vi "Write Lines.vi"(8 "error in (no error)":errorcluster, 10 "Lines":T1[](array[typedef]), 11 "J1939 configuration in":refnum<class "J1939 configuration.lvclass">) -> (0 "error out":errorcluster, 3 "J1939 configuration out":refnum<class "J1939 configuration.lvclass">)   [LabVIEW 2014, in "J1939 configuration.lvclass"]
uses:
  J1939 configuration.lvclass
  Line.ctl
  <vilib>/NI/Tag Bus Module Framework/channel/TBM channel.lvclass
  J1939 configuration.lvclass/J1939 configuration.ctl
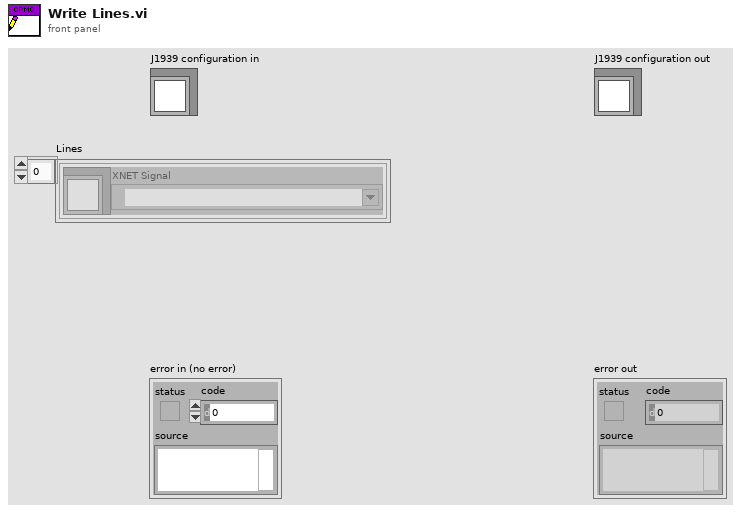
[diagram p1: front panel]
types:
  T1 = typedef "J1939 configuration.lvclass/Line.ctl" = cluster{"channel":refnum<class "TBM channel.lvclass">, "XNET Signal":refnum<k21>}
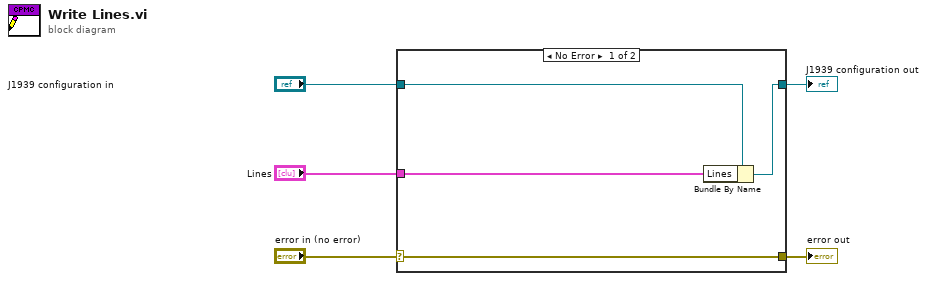
[diagram p0: block diagram]
diagram:
  n1 = case shown="No Error" "error in (no error)" {
    selector: "error in (no error)" -> [w9 w10]
    tunnel: [w9 w10] -> w4
    tunnel: [w7 w11] -> w2
    tunnel: "J1939 configuration in" -> [w8 w11]
    tunnel: "Lines" -> [w6 _]
    frame No Error {
      n2 = Bundle By Name(cluster=w8, "Lines"=w6) -> (w7:refnum<class "J1939 configuration.lvclass">)
    }
    frame Error {
    }
  }
  "error out" <- w4
  "J1939 configuration out" <- w2
